vi "Service Mode Entry.vi"(0 "GEA2 Reference In":refnum<k24>, 5 "Model":enum16{"HE", "LE"}(ring), 11 "Error In":errorcluster) -> (4 "GEA2 Reference Out":refnum<k24>, 6 "Pass/Fail?":bool, 8 "Report Text":string, 15 "Error Out":errorcluster)   [LabVIEW 2016, in "TLMB.lvlib"]
doc: "Use this VI to enter service mode."
uses:
  Projects/TLMB.lvlib
  Q:/Common/DLLs/GEA3/GeaCommunication.dll
  Common/DLLs/GEA3/GeaCommunication.dll
  Common/LabVIEW GEA2 Toolkit/LabVIEW_GEA2_Toolkit.lvlibp/type defs/Source_Destination.ctl
  Common/LabVIEW GEA2 Toolkit/LabVIEW_GEA2_Toolkit.lvlibp/type defs/ERD Read Data In.ctl
  Common/LabVIEW GEA2 Toolkit/LabVIEW_GEA2_Toolkit.lvlibp/type defs/Data Type.ctl
  type defs/Encoder Position.ctl
  Common/LabVIEW GEA2 Toolkit/LabVIEW_GEA2_Toolkit.lvlibp/type defs/ERD Write Data In.ctl
  Common/LabVIEW GEA2 Toolkit/LabVIEW_GEA2_Toolkit.lvlibp
panel:
  in  "Standalone?":bool
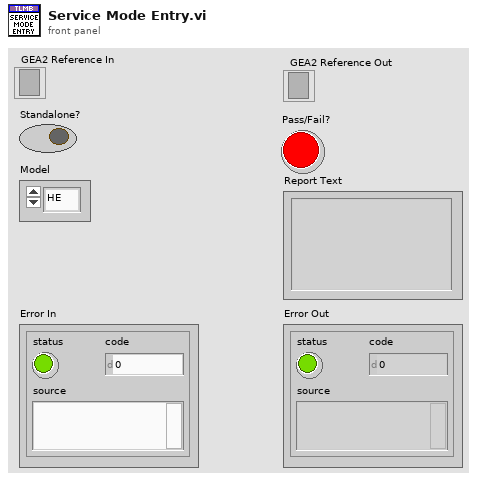
[diagram p1: front panel]
types:
  T1 = typedef "LabVIEW_GEA2_Toolkit.lvlibp/ERD Read Data In.ctl" = cluster{"ERD Number":u16, "Data Type":T2}
  T2 = typedef "LabVIEW_GEA2_Toolkit.lvlibp/Data Type.ctl" = enum16{"string", "boolean", "uint8_t", "uint16_t", "uint32_t", "uint64_t", "int8_t", "int16_t", "int32_t", "int64_t"}
  T3 = typedef "LabVIEW_GEA2_Toolkit.lvlibp/Source_Destination.ctl" = cluster{"Source":u8, "Destination":u8}
  T4 = typedef "LabVIEW_GEA2_Toolkit.lvlibp/ERD Write Data In.ctl" = cluster{"ERD Number":u16, "Data Type":T2, "Data":string}
  T5 = typedef "TLMB.lvlib/Encoder Position.ctl" = enum16{"Position 0", "Position 1", "Position 2", "Position 3", "Position 4", "Position 5", "Position 6", "Position 7", "Position 8", "Position 9", "Position 10", "Position 11", "Position 12", "Position 13", "Clear / Reset"}
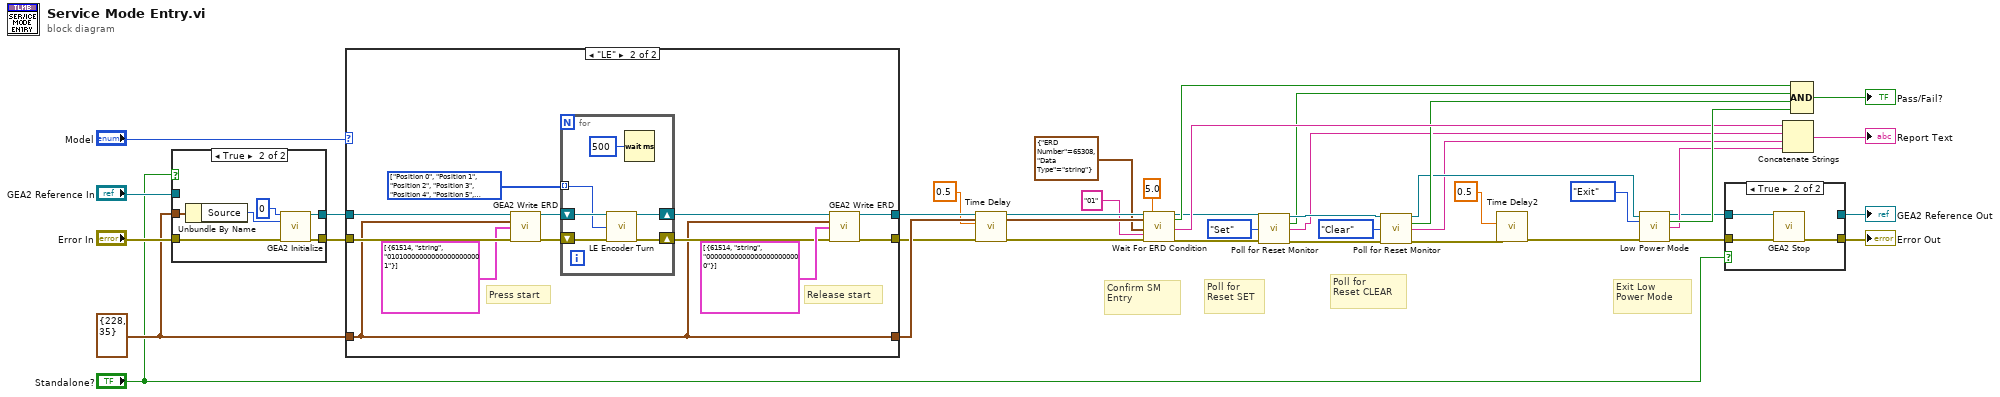
[diagram p0: block diagram]
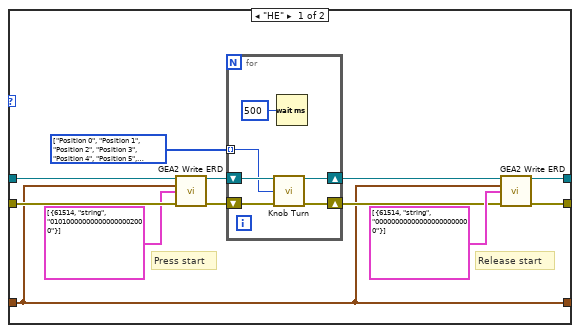
[diagram p2: hidden frame]
diagram:
  w34 = T3 {"Source"=228, "Destination"=35} ("GEA Inputs")
  # "Confirm SM \nEntry"
  # "Exit Low \nPower Mode"
  # "Poll for\nReset CLEAR"
  # "Poll for\nReset SET"
  n1 = case shown="True" "Standalone?" {
    tunnel: "Error In" -> [w41 w48]
    tunnel: [w41 w47] -> w36
    tunnel: "GEA2 Reference In" -> [w42 _]
    tunnel: [w42 w46] -> w37
    tunnel: w34 -> [_ w44]
    frame False {
    }
    frame True {
      n2 = Unbundle By Name(w44) -> ("Source"=w45:u8)
      n3 = call "GEA2 Initialize.vi"("Board Index"=0, "Source Address"=w45, "error in"=w48) -> ("GEA2 Reference Out"=w46:refnum<k24>, "error out"=w47:errorcluster)  [unwired: 10 in, 1 out]
    }
  }
  n4 = case shown="\"LE\"" "Model" {
    tunnel: w37 -> [w57 w75]
    tunnel: w36 -> [w56 w74]
    tunnel: w34 -> [w49 w67]
    tunnel: [w51 w69] -> w33
    tunnel: [w50 w68] -> w31
    tunnel: [w49 w67] -> w32
    frame "HE" {
      w60 = T5[] [enum."Position 0", enum."Position 1", enum."Position 2", enum."Position 3", enum."Position 4", enum."Position 5", enum."Position 6", enum."Position 7"] items=["Position 0", "Position 1", "Position 2", "Position 3", "Position 4", "Position 5", "Position 6", "Position 7", "Position 8", "Position 9", "Position 10", "Position 11", "Position 12", "Position 13", "Clear / Reset"]
      # "Release start"
      # "Press start"
      n5 = call "GEA2 Write ERD.vi"("GEA2 Reference In"=w57, "GEA Inputs"=w49, "Write ERD List"=T4[] [{"ERD Number"=61514, "Data Type"=enum."string", "Data"="010100000000000000002000"}], "Error In"=w56) -> ("GEA2 Reference Out"=w59:refnum<k24>, "Error Out"=w58:errorcluster)  [unwired: 9 in, 1 out]
      n6 = for {
        shift-right: [w65] -> w52
        shift-left: w59 -> [w66]
        shift-right: [w63] -> w53
        shift-left: w58 -> [w64]
        tunnel: w60 -> [w62] mode=indexing
        n7 = call "Knob Turn.vi"("GEA2 Reference In"=w66, "Knob Postiton"=w62, "Error In"=w64) -> ("GEA2 Reference Out"=w65:refnum<k24>, "Error Out"=w63:errorcluster)  [unwired: 11 in]
        n8 = Wait (ms)(milliseconds to wait=u32 500) -> ()  [unwired: 1 out]
      }
      n9 = call "GEA2 Write ERD.vi"("GEA2 Reference In"=w52, "GEA Inputs"=w49, "Write ERD List"=T4[] [{"ERD Number"=61514, "Data Type"=enum."string", "Data"="000000000000000000000000"}], "Error In"=w53) -> ("GEA2 Reference Out"=w51:refnum<k24>, "Error Out"=w50:errorcluster)  [unwired: 9 in, 1 out]
    }
    frame "LE" {
      w78 = T5[] [enum."Position 0", enum."Position 1", enum."Position 2", enum."Position 3", enum."Position 4", enum."Position 5", enum."Position 6", enum."Position 7"] items=["Position 0", "Position 1", "Position 2", "Position 3", "Position 4", "Position 5", "Position 6", "Position 7", "Position 8", "Position 9", "Position 10", "Position 11", "Position 12", "Position 13", "Clear / Reset"]
      # "Release start"
      # "Press start"
      n10 = call "GEA2 Write ERD.vi"("GEA2 Reference In"=w75, "GEA Inputs"=w67, "Write ERD List"=T4[] [{"ERD Number"=61514, "Data Type"=enum."string", "Data"="010100000000000000000001"}], "Error In"=w74) -> ("GEA2 Reference Out"=w77:refnum<k24>, "Error Out"=w76:errorcluster)  [unwired: 9 in, 1 out]
      n11 = for {
        shift-right: [w83] -> w70
        shift-left: w77 -> [w84]
        shift-right: [w81] -> w71
        shift-left: w76 -> [w82]
        tunnel: w78 -> [w80] mode=indexing
        n12 = call "LE Encoder Turn.vi"("GEA2 Reference In"=w84, "Button"=w80, "Error In"=w82) -> ("GEA2 Reference Out"=w83:refnum<k24>, "Error Out"=w81:errorcluster)  [unwired: 11 in]
        n13 = Wait (ms)(milliseconds to wait=u32 500) -> ()  [unwired: 1 out]
      }
      n14 = call "GEA2 Write ERD.vi"("GEA2 Reference In"=w70, "GEA Inputs"=w67, "Write ERD List"=T4[] [{"ERD Number"=61514, "Data Type"=enum."string", "Data"="000000000000000000000000"}], "Error In"=w71) -> ("GEA2 Reference Out"=w69:refnum<k24>, "Error Out"=w68:errorcluster)  [unwired: 9 in, 1 out]
    }
  }
  n15 = call "Time Delay"("error in (no error)"=w31, "Delay Time (s)"=0.5) -> ("error out"=w17:errorcluster)  [unwired: 9 in]
  n16 = call "Wait For ERD Condition.vi"("GEA2 Reference In"=w33, "GEA Inputs"=w32, "ERD Read Data"=T1 {"ERD Number"=65308, "Data Type"=enum."string"} ("ERD Read Data In"), "Expected Low"="01", "Error In"=w17, "Timeout (s)"=5.0) -> ("GEA2 Reference Out"=w7:refnum<k24>, "Pass/Fail?"=w18:bool, "Report Text"=w19:string, "Error Out"=w11:errorcluster)  [unwired: 9 in, 1 out]
  n17 = call "Poll for Reset Monitor.vi"("GEA2 Reference In"=w7, "Status"=enum16{"Clear", "Set"}."Set", "Error In"=w11) -> ("GEA2 Reference Out"=w6:refnum<k24>, "Pass/Fail?"=w5:bool, "Report Text"=w2:string, "Error Out"=w12:errorcluster)  [unwired: 8 in, 1 out]
  n18 = call "Poll for Reset Monitor.vi"("GEA2 Reference In"=w6, "Status"=enum16{"Clear", "Set"}."Clear", "Error In"=w12) -> ("GEA2 Reference Out"=w3:refnum<k24>, "Pass/Fail?"=w4:bool, "Report Text"=w1:string, "Error Out"=w10:errorcluster)  [unwired: 8 in, 1 out]
  n19 = call "Time Delay2"("error in (no error)"=w10, "Delay Time (s)"=0.5) -> ("error out"=w13:errorcluster)  [unwired: 9 in]
  n20 = call "Low Power Mode.vi"("GEA2 Reference In"=w3, "Action"=enum16{"Enter", "Exit"}."Exit", "Error In"=w13) -> ("GEA2 Reference Out"=w21:refnum<k24>, "Pass/Fail?"=w25:bool, "Report Text"=w24:string, "Error Out"=w26:errorcluster)  [unwired: 9 in]
  n21 = case shown="True" "Standalone?" {
    tunnel: [w86 w89] -> w40
    tunnel: w26 -> [w86 w88]
    tunnel: w21 -> [w85 w87]
    tunnel: [w85 _] -> w20
    frame False {
    }
    frame True {
      n22 = call "GEA2 Stop.vi"("GEA2 Reference In"=w87, "Error In"=w88) -> ("Error Out"=w89:errorcluster)  [unwired: 13 in]
    }
  }
  "Error Out" <- w40
  "GEA2 Reference Out" <- w20
  n23 = Concatenate Strings(w19, w2, w1, w24) -> (→"Report Text":string)
  n24 = Compound Arithmetic op=AND(w18, w5, w4, w25) -> (→"Pass/Fail?":bool)
